vi "Get Column Count.vi"(8 "error in (no error)":errorcluster, 11 "SQL Statement in":refnum<class "SQL Statement.lvclass">) -> (0 "error out":errorcluster, 2 "Number of Columns":i32, 3 "SQL Statement out":refnum<class "SQL Statement.lvclass">)   [LabVIEW 2011, in "SQLite.lvlib" / "SQL Statement.lvclass"]
doc: "Return the number of columns in the result set returned by the prepared statement. This routine returns 0 for an SQL statement that does not return data (for example an UPDATE)."
uses:
  SQL Statement.lvclass
  SQL Statement.lvclass/SQL Statement.ctl
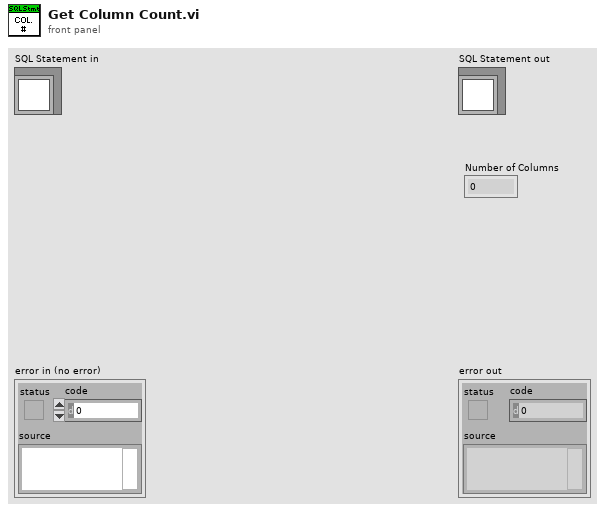
[diagram p1: front panel]
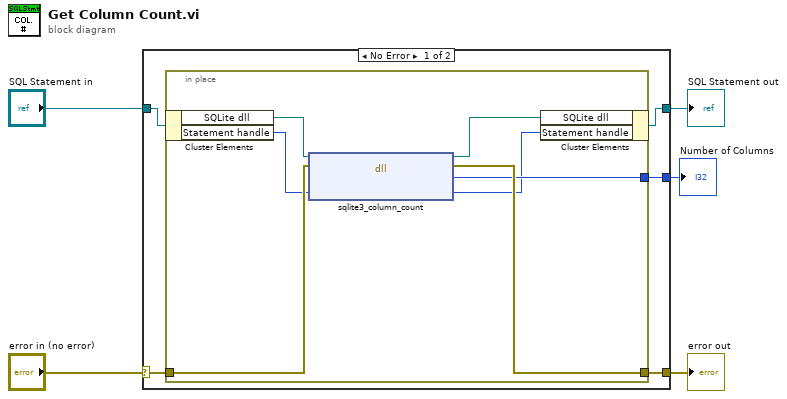
[diagram p0: block diagram]
diagram:
  n1 = case shown="No Error" "error in (no error)" {
    selector: "error in (no error)" -> [w10 w19]
    tunnel: [w9 w19] -> w4
    tunnel: [w6 w18] -> w2
    tunnel: "SQL Statement in" -> [w7 w18]
    tunnel: [w8 _] -> w1
    frame No Error {
      n2 = in-place {
        in-place-border: w10 -> [w17]
        in-place-border: [w16] -> w9
        in-place-border: [w15] -> w8
        n3 = in-place-cluster #1(w7) -> ("SQLite dll"=w14:path, "Statement handle"=w13:u64)
        n4 = dll-call lib="C:/SQLite/sqlite3.dll" fn="sqlite3_column_count"(path in=w14, error in=w17, "Statement"=w13) -> (path out=w11:path, error out=w16:errorcluster, "Number of Columns"=w15:i32, "Statement"=w12:u64)  [unwired: 1 in]
        n5 = in-place-cluster #1("SQLite dll"=w11, "Statement handle"=w12) -> (w6:refnum<class "SQL Statement.lvclass">)
      }
    }
    frame Error {
    }
  }
  "error out" <- w4
  "SQL Statement out" <- w2
  "Number of Columns" <- w1
